vi "ConfigureDataEventProperties.vi"(4 "default data block length":dbl, 6 "max time (sec)":dbl, 9 "channels":T1[](array[typedef]), 10 "group properties":T2[](array[typedef]), 11 "operating state":T4) -> (2 "AcqParams":T7)   [LabVIEW 2017, in "McsaDataEventCreator.lvlib"]
uses:
  <vilib>/addons/InsightCM/Devices/Shared/Mcsa/McsaDataEventCreator/McsaDataEventCreator.lvlib
  <vilib>/addons/InsightCM/Devices/Shared/Mcsa/McsaDataEventCreator/controls/AcqParams.ctl
  <vilib>/addons/InsightCM/Devices/Shared/Common/DataAccumulator/controls/AccumulationSettings.ctl
  <vilib>/addons/InsightCM/Devices/Shared/Common/DataAccumulator/controls/accumulationType.ctl
  <vilib>/addons/InsightCM/Devices/Shared/Common/DVRBuffer/controls/BufferLocation.ctl
  <vilib>/addons/InsightCM/MessageBus/Base/controls/OperatingState.ctl
  <vilib>/addons/InsightCM/MessageBus/Base/controls/KeyValuePair.ctl
  <vilib>/addons/InsightCM/MessageBus/Base/controls/Trigger.ctl
  <vilib>/addons/InsightCM/MessageBus/Base/controls/Condition.ctl
  <vilib>/addons/InsightCM/MessageBus/Base/controls/R2_Channel.ctl
  <vilib>/addons/InsightCM/MessageBus/Base/controls/Metric.ctl
  <vilib>/addons/InsightCM/Utilities/PropertyHelpers/PropertyHelpers.lvlib
  <vilib>/addons/InsightCM/Devices/Shared/Common/DVRBuffer/DVRBuffer.lvlib
  <vilib>/addons/InsightCM/Devices/Shared/Common/DataAccumulator/DataAccumulator.lvlib
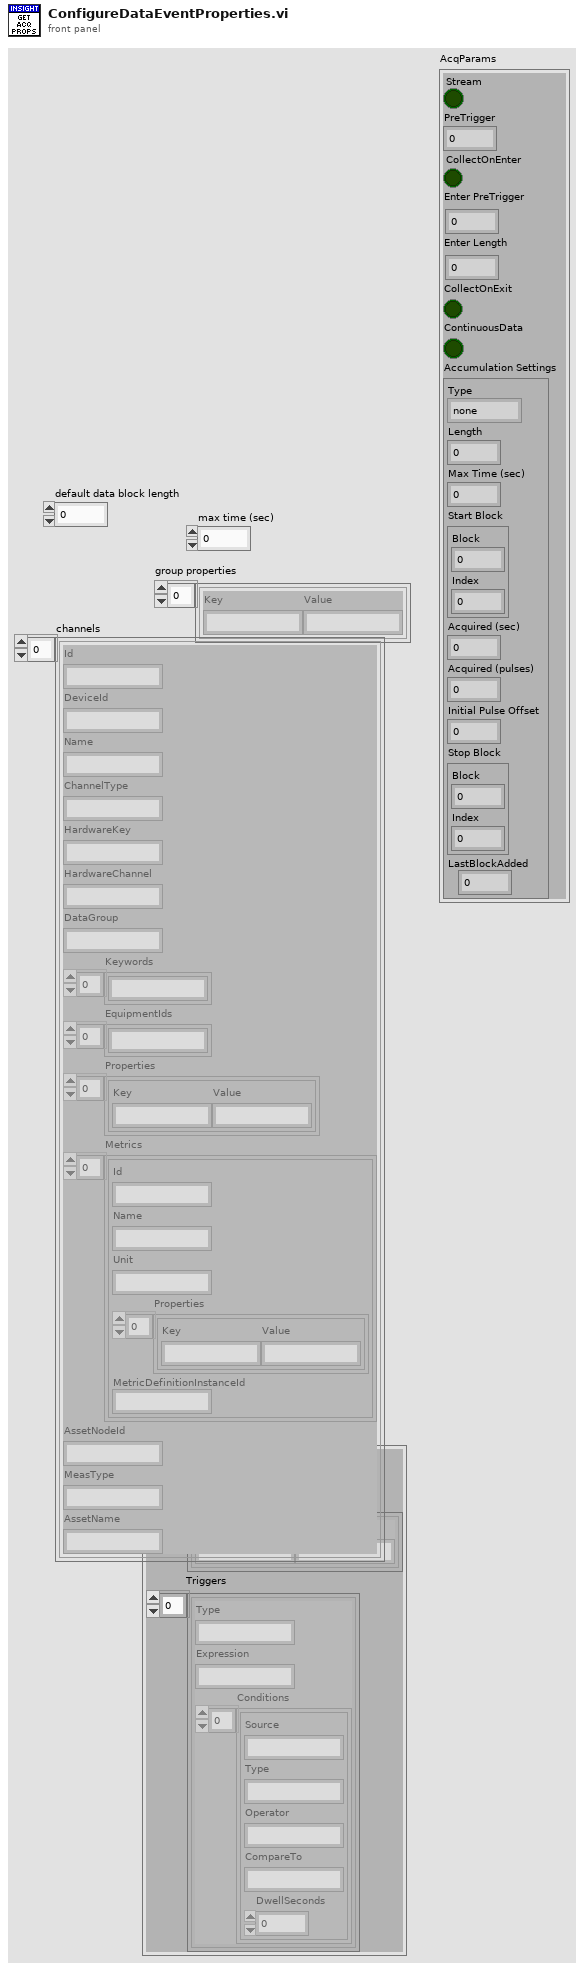
[diagram p1: front panel]
types:
  T1 = typedef "R2_Channel.ctl" = cluster{"Id":string, "DeviceId":string, "Name":string, "ChannelType":string, "HardwareKey":string, "HardwareChannel":string, "DataGroup":string, "Keywords":string[], "EquipmentIds":string[], "Properties":T2[], "Metrics":T3[], "AssetNodeId":string, "MeasType":string, "AssetName":string}
  T2 = typedef "KeyValuePair.ctl" = cluster{"Key":string, "Value":string}
  T3 = typedef "Metric.ctl" = cluster{"Id":string, "Name":string, "Unit":string, "Properties":T2[], "MetricDefinitionInstanceId":string}
  T4 = typedef "OperatingState.ctl" = cluster{"Name":string, "Properties":T2[], "Triggers":T5[]}
  T5 = typedef "Trigger.ctl" = cluster{"Type":string, "Expression":string, "Conditions":T6[]}
  T6 = typedef "Condition.ctl" = cluster{"Source":string, "Type":string, "Operator":string, "CompareTo":string, "DwellSeconds":dbl}
  T7 = typedef "McsaDataEventCreator.lvlib/AcqParams.ctl" = cluster{"Stream":bool, "PreTrigger":i32, "CollectOnEnter":bool, "Enter PreTrigger":i32, "Enter Length":dbl, "CollectOnExit":bool, "ContinuousData":bool, "Accumulation Settings":T8}
  T8 = typedef "DataAccumulator.lvlib/AccumulationSettings.ctl" = cluster{"Type":T9, "Length":dbl, "Max Time (sec)":dbl, "Start Block":T10, "Acquired (sec)":dbl, "Acquired (pulses)":i32, "Initial Pulse Offset":dbl, "Stop Block":T10, "LastBlockAdded":u32}
  T9 = typedef "DataAccumulator.lvlib/accumulationType.ctl" = enum16{"none", "seconds", "revolutions"}
  T10 = typedef "DVRBuffer.lvlib/BufferLocation.ctl" = cluster{"Block":u32, "Index":i32}
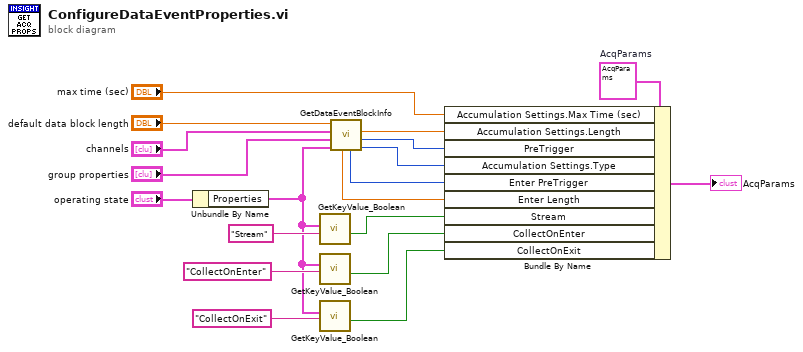
[diagram p0: block diagram]
diagram:
  w14 = T7 {"Stream"=FALSE, "PreTrigger"=0, "CollectOnEnter"=FALSE, "Enter PreTrigger"=0, "Enter Length"=0.0, "CollectOnExit"=FALSE, "ContinuousData"=FALSE, "Accumulation Settings"={"Type"=enum."none", "Length"=0.0, "Max Time (sec)"=0.0, "Start Block"={"Block"=0, "Index"=0}, "Acquired (sec)"=0.0, "Acquired (pulses)"=0, "Initial Pulse Offset"=0.0, "Stop Block"={"Block"=0, "Index"=0}, "LastBlockAdded"=0}}  # AcqParams
  n1 = Unbundle By Name("operating state") -> ("Properties"=w5:T2[])
  n2 = call <vilib>:"GetKeyValue_Boolean.vi"("key"="Stream", "key value pairs"=w5) -> ("value"=w4:bool)  [unwired: 7 in, 2 out]
  n3 = call <vilib>:"GetKeyValue_Boolean.vi"("key"="CollectOnEnter", "key value pairs"=w5) -> ("value"=w15:bool)  [unwired: 7 in, 2 out]
  n4 = call <vilib>:"GetKeyValue_Boolean.vi"("key"="CollectOnExit", "key value pairs"=w5) -> ("value"=w6:bool)  [unwired: 7 in, 2 out]
  n5 = call <vilib>:"GetDataEventBlockInfo.vi"("operating state properties"=w5, "group properties"="group properties", "channels"="channels", "default data block length"="default data block length") -> ("type"=w8:T9, "pritrigger"=w10:i32, "total length"=w9:dbl, "enter pretrigger"=w3:i32, "enter total length"=w2:dbl)  [unwired: 2 in, 1 out]
  n6 = Bundle By Name(cluster=w14, "Accumulation Settings.Max Time (sec)"="max time (sec)", "Accumulation Settings.Length"=w9, "PreTrigger"=w10, "Accumulation Settings.Type"=w8, "Enter PreTrigger"=w3, "Enter Length"=w2, "Stream"=w4, "CollectOnEnter"=w15, "CollectOnExit"=w6) -> (→"AcqParams":T7)
